vi "EditorMethod runGraphProcess.vi"(5 "xyGraphRefnum":refnum<vi>, 7 "state":T1, 8 "error in (no error)":errorcluster, 9 "This VI":refnum<vi>, 10 "currFilePath":path, 11 "signal in":waveform(sgl)) -> (0 "error out":errorcluster)   [LabVIEW 2018]
uses:
  ctl/dataGraphState.ctl
  ctl/dataListboxState.ctl
  PC/PublicSubVI/Class/Sig2MS/Sig2MS.lvclass
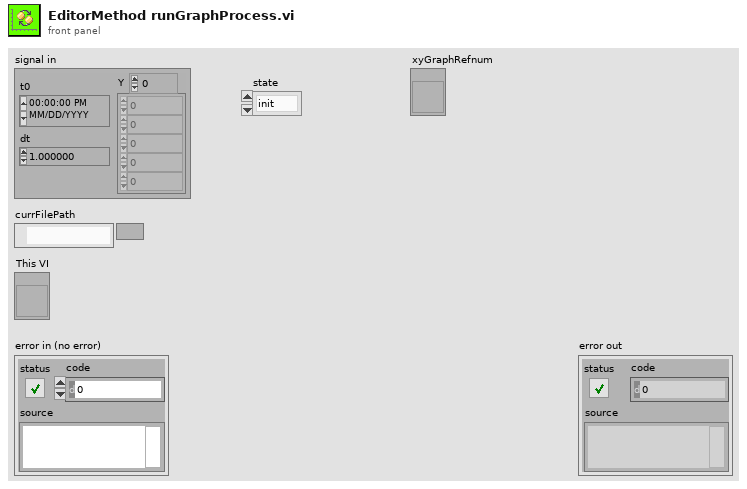
[diagram p1: front panel]
types:
  T1 = typedef "dataGraphState.ctl" = enum16{"init", "set"}
  T2 = typedef "dataListboxState.ctl" = enum16{"init", "setData", "upd", "getExport"}
  T3 = cluster{"startTime":dbl, "scanSig":cluster{"priDt":dbl, "priXData":dbl[], "priYData":sgl[], "beta":dbl[]}[]}
  T4 = cluster{"startTime":dbl, "scanSig":cluster{"priDt":dbl, "priXData":dbl[], "priYData":sgl[], "beta":dbl[]}[], "ionSig":cluster{"secDt":dbl, "secYData":sgl[]}[]}
  T5 = cluster{"priDt":dbl, "priXData":dbl[], "priYData":sgl[], "beta":dbl[]}[]
  T6 = cluster{"startTime":dbl, "scanData":cluster{"dt":dbl, "xdata":dbl[], "ydata":sgl[], "beta":dbl[]}[], "xyXLabel":string, "xyYLabel":string, "peakData":cluster{"xLeftIdx":u32[], "xCenterIdx":u32[], "xRightIdx":u32[], "baseline":sgl[], "halfHeight":dbl[]}[]}
  T7 = cluster{"dt":dbl, "xdata":dbl[], "ydata":sgl[], "beta":dbl[]}[]
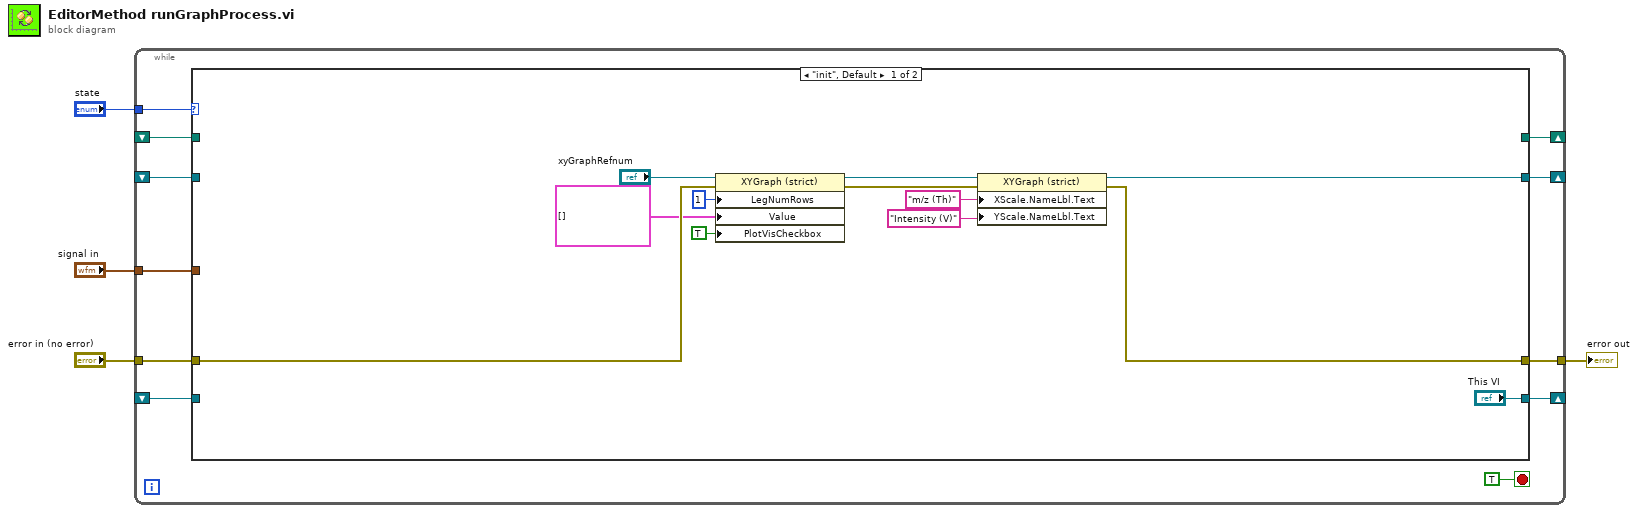
[diagram p0: block diagram]
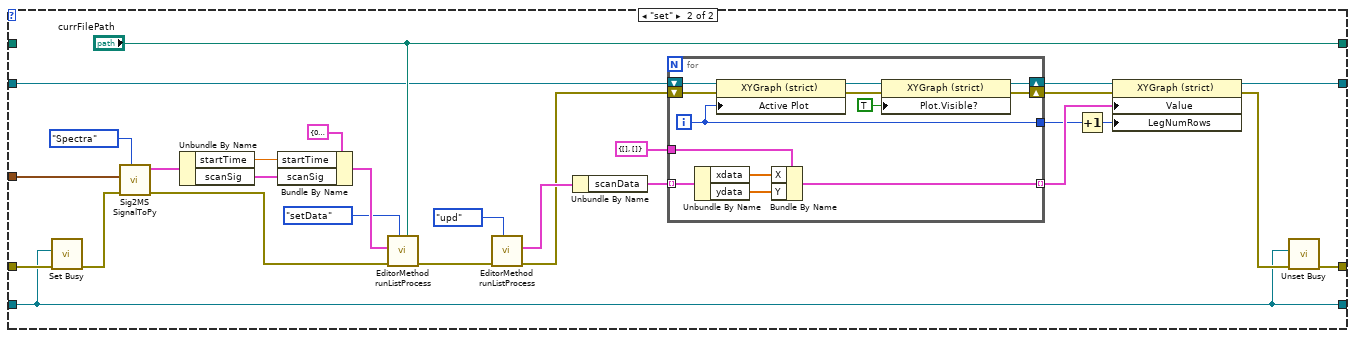
[diagram p2: hidden frame]
diagram:
  n1 = while {
    tunnel: "state" -> [w15]
    shift-right: [w14] -> _
    shift-left: _ -> [w13]
    tunnel: "signal in" -> [w12]
    shift-right: [w10] -> _
    shift-left: _ -> [w9]
    tunnel: "error in (no error)" -> [w8]
    tunnel: [w7] -> w1
    shift-right: [w5] -> _
    shift-left: _ -> [w6]
    stop <- TRUE stop-if-true
    n2 = case shown="\"init\", Default" w15 {
      tunnel: [w21 w53] -> w14
      tunnel: w13 -> [_ w30]
      tunnel: w12 -> [_ w54]
      tunnel: [_ "currFilePath"] -> w10
      tunnel: w9 -> [_ _]
      tunnel: w8 -> [w20 w38]
      tunnel: [w19 w35] -> w7
      tunnel: w6 -> [_ w34]
      tunnel: ["This VI" w34] -> w5
      frame "init", Default {
        n3 = property class="XYGraph (strict)"(reference="xyGraphRefnum", error in=w20, "LegNumRows"=u32 1 ("Legend:Number of Rows"), "Value"=cluster{"X":dbl[], "Y":sgl[]}[] [], "PlotVisCheckbox"=TRUE ("Legend:Plot Visibility Checkbox Visible")) -> (reference out=w25:refnum<vi>, error out=w24:errorcluster)
        n4 = property class="XYGraph (strict)"(reference=w25, error in=w24, "XScale.NameLbl.Text"="m/z (Th)" ("X Scale.Name Label.Text"), "YScale.NameLbl.Text"="Intensity (V)" ("Y Scale.Name Label.Text")) -> (reference out=w21:refnum<vi>, error out=w19:errorcluster)
      }
      frame "set" {
        n5 = call <vilib>:"Set Busy.vi"("error in (no error)"=w38, "VI reference (current VI)"=w34) -> ("error out"=w37:errorcluster)  [unwired: 8 in, 1 out]
        n6 = call "Sig2MS SignalToPy.vi"("getType"=enum16{"All", "Spectra", "Ionisation"}."Spectra", "error in (no error)"=w37, "rawSignal"=w54) -> ("error out"=w42:errorcluster, "pySigFormat"=w49:T4)  [unwired: 7 in]
        n7 = Unbundle By Name(w49) -> ("startTime"=w47:dbl, "scanSig"=w46:T5)
        n8 = Bundle By Name(cluster=T3 {"startTime"=0.0, "scanSig"=[]} ("dataParam"), "startTime"=w47, "scanSig"=w46) -> (w45:T3)
        n9 = call "EditorMethod runListProcess.vi"("currFilePath"="currFilePath", "state"=dataListboxState."setData", "error in (no error)"=w42, "dataParam"=w45) -> ("error out"=w41:errorcluster)  [unwired: 4 in, 3 out]
        n10 = call "EditorMethod runListProcess.vi"("state"=dataListboxState."upd", "error in (no error)"=w41) -> ("error out"=w29:errorcluster, "newSigInfo"=w39:T6)  [unwired: 6 in, 2 out]
        n11 = Unbundle By Name(w39) -> ("scanData"=w52:T7)
        n12 = for {
          tunnel: w52 -> [w68] mode=indexing
          tunnel: cluster{"X":dbl[], "Y":sgl[]} {"X"=[], "Y"=[]} ("Spectrum in") -> [w67]
          tunnel: [w64] -> w50 mode=indexing
          tunnel: [w62] -> w33
          shift-right: [w60] -> w31
          shift-left: w30 -> [w63]
          shift-right: [w56] -> w28
          shift-left: w29 -> [w57]
          i -> [w62]
          n13 = Unbundle By Name(w68) -> ("xdata"=w66:dbl[], "ydata"=w65:sgl[])
          n14 = property class="XYGraph (strict)"(reference=w63, error in=w57, "Active Plot"=w62) -> (reference out=w61:refnum<vi>, error out=w58:errorcluster)
          n15 = Bundle By Name(cluster=w67, "X"=w66, "Y"=w65) -> (w64:cluster{"X":dbl[], "Y":sgl[]})
          n16 = property class="XYGraph (strict)"(reference=w61, error in=w58, "Plot.Visible?"=TRUE ("Plot.Visible")) -> (reference out=w60:refnum<vi>, error out=w56:errorcluster)
        }
        n17 = Increment(x=w33) -> (x+1=w32:i32)
        n18 = property class="XYGraph (strict)"(reference=w31, error in=w28, "Value"=w50, "LegNumRows"=w32) -> (reference out=w53:refnum<vi>, error out=w36:errorcluster)
        n19 = call <vilib>:"Unset Busy.vi"("error in (no error)"=w36, "VI reference (current VI)"=w34) -> ("error out"=w35:errorcluster)  [unwired: 9 in]
      }
    }
  }
  "error out" <- w1
